vi "PixieUserPar.vi"(7 "ModNum":u16, 8 "error in (no error)":errorcluster, 9 "ChanNum":u16, 10 "User_Par_Type":string, 11 "User_Par_Name":string) -> (0 "error out":errorcluster, 2 "User_Par_Value":dbl)   [LabVIEW 2013]
doc: "Use this template to build a VI to use as a subVI."
uses:
  XIA/Pixie4/Drivers/Pixie4DLL.dll
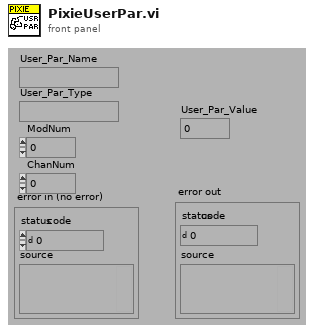
[diagram p1: front panel]
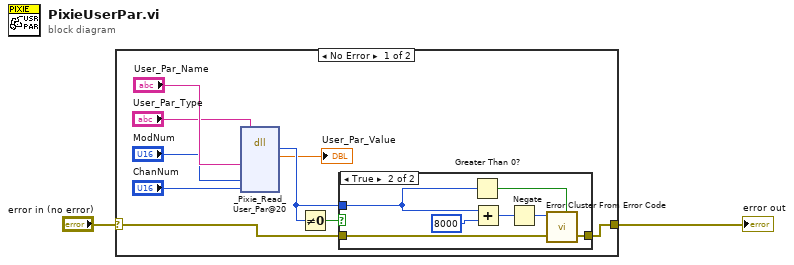
[diagram p0: block diagram]
diagram:
  n1 = case shown="No Error" "error in (no error)" {
    selector: "error in (no error)" -> [w10 w20]
    tunnel: [w11 w20] -> w1
    frame No Error {
      n2 = dll-call lib="C:/XIA/Pixie4/Drivers/Pixie4DLL.dll" fn="_Pixie_Read_User_Par@20"("User_Par_Name"="User_Par_Name", "User_Par_Type"="User_Par_Type", "ModNum"="ModNum", "ChanNum"="ChanNum") -> ("return type"=w8:i32, "User_Par_Value"=→"User_Par_Value":dbl)  [unwired: 7 in, 3 out]
      n3 = Not Equal To 0?(x=w8) -> (x != 0?=w9:bool)
      n4 = case shown="True" w9 {
        tunnel: w8 -> [_ w19]
        tunnel: [w12 w14] -> w11
        tunnel: w10 -> [w12 w13]
        frame False {
        }
        frame True {
          n5 = Greater Than 0?(x=w19) -> (x > 0?=w16:bool)
          n6 = Add(x=w19, y=8000) -> (x+y=w17:i32)
          n7 = Negate(x=w17) -> (-x=w15:i32)
          n8 = call <vilib>:"Error Cluster From Error Code.vi"("is warning? (False)"=w16, "error in (no error)"=w13, "error code (0)"=w15) -> ("error out"=w14:errorcluster)  [unwired: 1 in, 5 out]
        }
      }
    }
    frame Error {
    }
  }
  "error out" <- w1
